vi "Calculator-setup.vi"(7 "test case ID":string) -> (1 "Y":dbl, 2 "X":dbl, 4 "Operation":T1)   [LabVIEW 2018]
uses:
  Code/Operation--enum.ctl
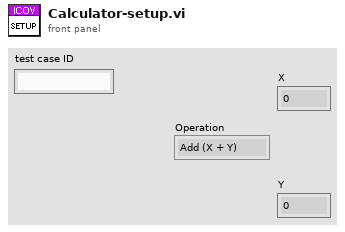
[diagram p1: front panel]
types:
  T1 = typedef "Operation--enum.ctl" = enum16{"Add (X + Y)", "Subtract (X - Y)", "Multiply (X * Y)", "Divide (X / Y)"}
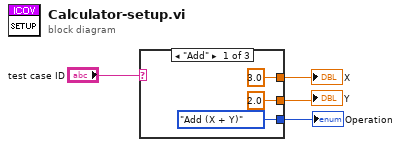
[diagram p0: block diagram]
diagram:
  n1 = case shown="\"Add\"" "test case ID" {
    tunnel: [3.0 ("X") _ _] -> w3
    tunnel: [2.0 ("Y") _ _] -> w2
    tunnel: [Operation--enum."Add (X + Y)" ("Operation") _ _] -> w1
    frame "Add" {
    }
    frame "testcaseID2" {
    }
    frame Default {
    }
  }
  "X" <- w3
  "Y" <- w2
  "Operation" <- w1
